vi "Drive Distance.vi"() -> ()   [LabVIEW 2016]
uses:
  Refname/Motors.ctl
  Refname/Refname to String (Motors).vi
panel:
  in  "Drive Angle":dbl
  in  "Drive Magnitude":dbl
  in  "Distance (inches)":dbl
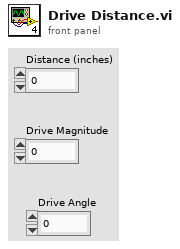
[diagram p1: front panel]
types:
  T1 = typedef "Motors.ctl" = enum16{"Wheel 1", "Swerve 1", "Wheel 2", "Swerve 2", "Wheel 3", "Swerve 3", "Wheel 4", "Swerve 4"}
  T2 = typedef "WPI_MotorControlDeviceRef.ctl" = cluster{"DeviceStatus":errorcluster, "Type":T3, "PWM":cluster{"PWM Channel":T4, "DeadBand":T5}, "CAN":cluster{"Device Number":u8, "SetOutput VI Ref":variant, "GetOutput VI Ref":variant, "Enable VI Ref":variant, "Disable VI Ref":variant, "Data":variant}, "Invert":bool}
  T3 = typedef "WPI_MotorControlType.ctl" = enum16{"PWM", "CAN"}
  T4 = typedef "FPGA_DIOPWMChannel.ctl" = enum8{"PWM 0", "PWM 1", "PWM 2", "PWM 3", "PWM 4", "PWM 5", "PWM 6", "PWM 7", "PWM 8", "PWM 9", "PWM MXP 0", "PWM MXP 1", "PWM MXP 2", "PWM MXP 3", "PWM MXP 4", "PWM MXP 5", "PWM MXP 6", "PWM MXP 7", "PWM MXP 8", "PWM MXP 9", "Invalid"}
  T5 = typedef "WPI_PWMDeadband.ctl" = cluster{"Name":string, "maxPositivePwm":i32, "minPositivePwm":i32, "centerPwm":i32, "maxNegativePwm":i32, "minNegativePwm":i32, "angularRange":u16}
  T6 = typedef "WPI_CANTalonSRX_GlobalStatus.ctl" = cluster{"Applied Throttle":dbl, "Module Enabled":bool, "CAN Error":errorcluster, "Closed Loop Error":dbl, "Forward Limit Switch Closed":bool, "Reverse Limit Switch Closed":bool, "Sensor Position":dbl, "Sensor Velocity":dbl, "Current":dbl, "Sticky Fault - Over Temp":bool, "Sticky Fault - Under Voltage":bool, "Sticky Fault - Forward Limit":bool, "Sticky Fault - Reverse Limit":bool, "Sticky Fault - Forward Soft Limit":bool, "Sticky Fault - Reverse Soft Limit":bool, "Brake is Enabled":bool, "Encoder Position":dbl, "Encoder Velocity":dbl, "Encoder Index Count":dbl, "Encoder A Pin State":bool, "Encoder B Pin State":bool, "Encoder Index Pin State":bool, "Analog In":dbl, "Analog In Velocity":dbl, "Temperature (C)":dbl, "Battery Voltage":dbl, "Control 5 Is Supported":bool, "Current Profile Slot Select":dbl, "Pos Div 8":bool, "Vel Div 4":bool, "Pulse Width Position":i32, "Pulse Width Velocity":i32, "Pulse Width Rise To Rise (us)":i32, "Pulse Width Rise To Fall (us)":i32, "Mot Prof Active Is Under Run":bool, "Mot Prof Active Has Under Run":bool, "Mot Prof Active Is Last":bool, "Mot Prof Active Velocity Only":bool, "Mot Prof Active Is Valid":bool, "Mot Prof Buffer Is Full":bool, "Mot Prof Active Profile Slot Select":i32, "Mot Prof NextID":i32, "Mot Prof Count":i32, "Mot Prof Active Velocity":dbl, "Mot Prof Active Position":dbl, "Mot Prof Output Enable":i32}
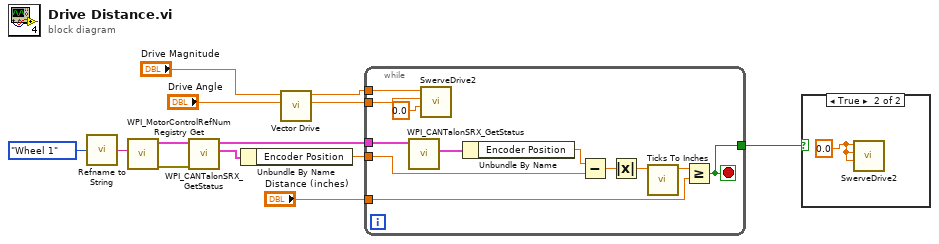
[diagram p0: block diagram]
diagram:
  n1 = call-poly "Refname to String.vi"("Enum"=Motors."Wheel 1") -> ("String"=w9:string)
  n2 = call <vilib>:"WPI_MotorControlRefNum Registry Get.vi"("refnum name"=w9) -> ("error out"=w8:errorcluster, "MotorControlDevRef"=w7:T2)  [unwired: 9 in]
  n3 = call <vilib>:"WPI_CANTalonSRX_GetStatus.vi"("error in (no error)"=w8, "CAN Talon SRX Ref"=w7) -> ("Talon SRX Status"=w6:T6, "CAN Talon SRX Ref"=w4:T2)  [unwired: 7 in, 1 out]
  n4 = Unbundle By Name(w6) -> ("Encoder Position"=w5:dbl)
  n5 = call "Vector Drive.vi"("Drive Angle"="Drive Angle", "Drive Magnitude"="Drive Magnitude") -> ("Forward"=w2:dbl, "Strafe"=w3:dbl)  [unwired: 7 in, 1 out]
  n6 = while {
    tunnel: "Distance (inches)" -> [w18]
    tunnel: w5 -> [w22]
    tunnel: w4 -> [w25]
    tunnel: w3 -> [w17]
    tunnel: w2 -> [w16]
    tunnel: [w14] -> w1
    stop <- w14 stop-if-true
    n7 = call <vilib>:"WPI_CANTalonSRX_GetStatus.vi"("CAN Talon SRX Ref"=w25) -> ("Talon SRX Status"=w24:T6)  [unwired: 8 in, 2 out]
    n8 = call "SwerveDrive2.vi"("Rotate"=0.0, "Forward"=w16, "Strafe"=w17) -> ()  [unwired: 8 in, 1 out]
    n9 = Unbundle By Name(w24) -> ("Encoder Position"=w23:dbl)
    n10 = Subtract(x=w23, y=w22) -> (x-y=w21:dbl)
    n11 = Absolute Value(x=w21) -> (abs(x)=w20:dbl)
    n12 = call "Ticks To Inches.vi"("Ticks"=w20) -> ("Inches"=w19:dbl)  [unwired: 9 in, 1 out]
    n13 = Greater Or Equal?(x=w19, y=w18) -> (x >= y?=w14:bool)
  }
  n14 = case shown="True" w1 {
    frame False {
    }
    frame True {
      w26 = 0.0 ("Rotate")
      n15 = call "SwerveDrive2.vi"("Rotate"=w26, "Forward"=w26, "Strafe"=w26) -> ()  [unwired: 8 in, 1 out]
    }
  }
